vi "AnalysatorInListeFinden.vi"(10 "AnalysatorDefinition":T1, 11 "AnalysatorListe":T1[](array[typedef])) -> (0 "gefunden":bool, 1 "Index":i32, 2 "AnalysatorDefinition out":T1, 3 "AnalysatorListe out":T1[](array[typedef]))   [LabVIEW 2020, in "System Einstellungen V2.lvlib"]
uses:
  System Einstellungen V2.lvlib
  AnalysatorDefinition.ctl
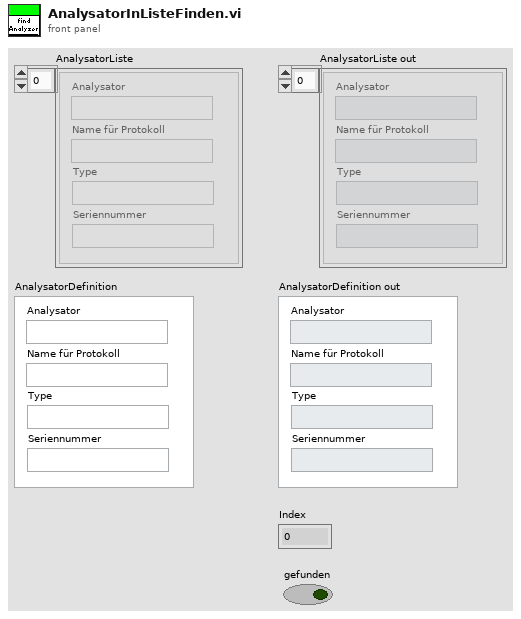
[diagram p1: front panel]
types:
  T1 = typedef "System Einstellungen V2.lvlib/AnalysatorDefinition.ctl" = cluster{"Analysator":string, "Name für Protokoll":string, "Type":string, "Seriennummer":string}
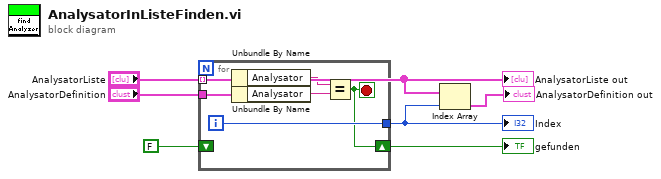
[diagram p0: block diagram]
diagram:
  n1 = for {
    tunnel: "AnalysatorDefinition" -> [w11]
    tunnel: "AnalysatorListe" -> [w12] mode=indexing
    tunnel: [w8] -> w2
    shift-right: [w7] -> w4
    shift-left: FALSE -> [_]
    i -> [w8]
    stop <- w7 stop-if-true
    n2 = Unbundle By Name(w12) -> ("Analysator"=w10:string)
    n3 = Unbundle By Name(w11) -> ("Analysator"=w9:string)
    n4 = Equal?(x=w10, y=w9) -> (x = y?=w7:bool)
  }
  "Index" <- w2
  "gefunden" <- w4
  n5 = Index Array(array="AnalysatorListe", index=w2) -> (element=→"AnalysatorDefinition out":T1)
  "AnalysatorListe out" <- "AnalysatorListe"
